vi "OpenCVCam_GetImage.vi"(8 "ErrorIn":errorcluster, 11 "OpenCVCamIn":refnum<class "OpenCVCam.lvclass">) -> (0 "ErrorOut":errorcluster, 2 "NewPicture":picture, 3 "OpenCVCamOut":refnum<class "OpenCVCam.lvclass">)   [LabVIEW 2021, in "OpenCVCam.lvclass"]
uses:
  OpenCVCam.lvclass
  OpenCVCam.lvclass/OpenCVCam.ctl
  C:/Localdata/Projects/TriekselSoft/TriekselsoftApplicationFramework/Source/.Externals/Library_EmguCV/Emgu.CV.Platform.NetStandard.dll
  .Externals/Library_EmguCV/Emgu.CV.Platform.NetStandard.dll
  .Externals/INewOpenCVMat/INewOpenCVMat.lvclass
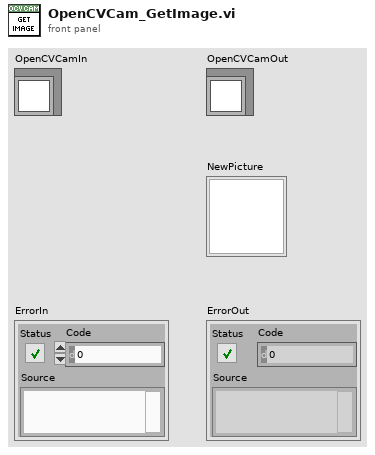
[diagram p1: front panel]
types:
  T1 = typedef "OpenCVCam.lvclass/State.ctl" = enum16{"Idle", "Initialized", "Acquiring"}
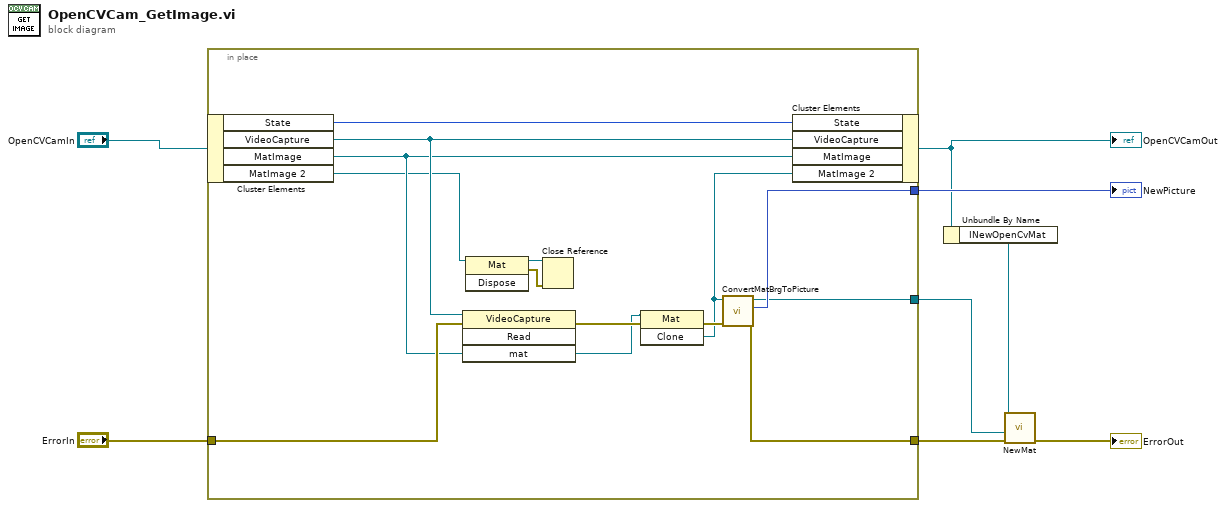
[diagram p0: block diagram]
diagram:
  n1 = in-place {
    in-place-border: "ErrorIn" -> [w21]
    in-place-border: [w20] -> w8
    in-place-border: [w14] -> w5
    in-place-border: [w13] -> w1
    n2 = in-place-cluster #1("OpenCVCamIn") -> ("State"=w15:T1, "VideoCapture"=w16:refnum<k24>, "MatImage"=w12:refnum<k24>, "MatImage 2"=w10:refnum<k24>)
    n3 = invoke class="VideoCapture" method="Read"(reference=w16, error in=w21, "mat"=w12) -> (error out=w19:errorcluster)  [unwired: 1 in, 3 out]
    n4 = invoke class="Mat" method="Dispose"(reference=w10) -> (reference out=w9:refnum<k24>, error out=w18:errorcluster)  [unwired: 2 in, 1 out]
    n5 = Close Reference(reference=w9, error in (no error)=w18) -> ()  [unwired: 1 out]
    n6 = invoke class="Mat" method="Clone"(reference=w12, error in=w19) -> (error out=w17:errorcluster, "Clone"=w11:refnum<k24>)  [unwired: 1 in, 1 out]
    n7 = call "ConvertMatBrgToPicture.vi"("ErrorIn"=w17, "CvMatIn"=w11) -> ("ErrorOut"=w20:errorcluster, "NewPicture"=w14:picture, "CvMatOut"=w13:refnum<k24>)  [unwired: 7 in]
    n8 = in-place-cluster #1("State"=w15, "VideoCapture"=w16, "MatImage"=w12, "MatImage 2"=w11) -> (w3:refnum<class "OpenCVCam.lvclass">)
  }
  "NewPicture" <- w5
  "OpenCVCamOut" <- w3
  n9 = Unbundle By Name(w3) -> ("INewOpenCvMat"=w2:refnum<class "INewOpenCVMat.lvclass">)
  n10 = call-dynamic "NewMat.vi"("ErrorIn"=w8, "CvMat"=w1, "ObjectIn"=w2) -> ("ErrorOut"=→"ErrorOut":errorcluster)  [unwired: 7 in, 1 out]
